vi "E16_GraficoIntensidad.vi"() -> ()   [LabVIEW 2026]
panel:
  out "Intensity Graph":dbl[][](graph)
  out "Array":dbl[][](array[numeric])
  in  "Columnas":i32
  in  "Filas":i32
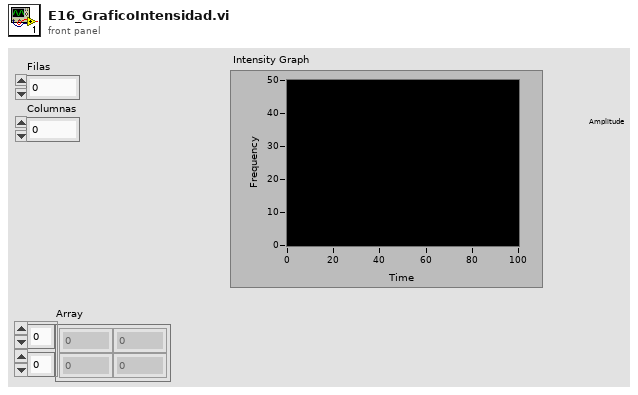
[diagram p1: front panel]
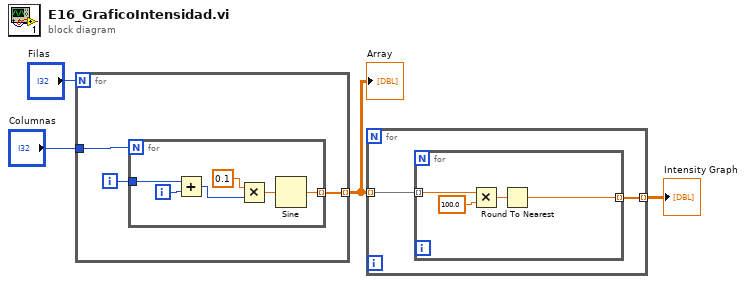
[diagram p0: block diagram]
diagram:
  n1 = for {
    N: "Filas" -> [_]
    tunnel: "Columnas" -> [w7]
    tunnel: [w5] -> w1 mode=indexing
    i -> [w6]
    n2 = for {
      N: w7 -> [_]
      tunnel: w6 -> [w12]
      tunnel: [w8] -> w5 mode=indexing
      i -> [w13]
      n3 = Add(x=w12, y=w13) -> (x+y=w11:i32)
      n4 = Multiply(x=0.1, y=w11) -> (x*y=w9:dbl)
      n5 = Sine(x=w9) -> (sin(x)=w8:dbl)
    }
  }
  "Array" <- w1
  n6 = for {
    tunnel: w1 -> [w15] mode=indexing
    tunnel: [w14] -> w2 mode=indexing
    n7 = for {
      tunnel: w15 -> [w19] mode=indexing
      tunnel: [w16] -> w14 mode=indexing
      n8 = Multiply(x=w19, y=100.0) -> (x*y=w17:dbl)
      n9 = Round To Nearest(number=w17) -> (nearest integer value=w16:dbl)
    }
  }
  "Intensity Graph" <- w2
